vi "Enforce array size one timestamp.vi"(9 "#bytes per timestamp":i32, 11 "Values (new)":u8[](array[numeric])) -> (3 "Values (new) [padded]":u8[](array[numeric]))   [LabVIEW 2021, in "Ring Buffer Time Series Data.lvlib"]
doc: "This VIM will set a size to the <b>Array In</b> and pass it out as <b>Array Out</b>. This VIM can set a Minimum, or Maximum array size setting <b>Mode</b>. The size is then specified with <b>Size</b>. If elements need to be added or removed they can be processed to at the start of the array or the end. Returned will be the elements that needed to be added or removed to meet the size needs.\n\n-------------\nPackage Information\n\nProduct Name: Hooovahh Array VIMs\nPackage File Name: Hooovahh_Array_VIMs-2.1.1.12\nPackage Version: 2.1.1.12\nMinimum LabVIEW Version: 18.0"
uses:
  Ring Buffer Time Series Data.lvlib
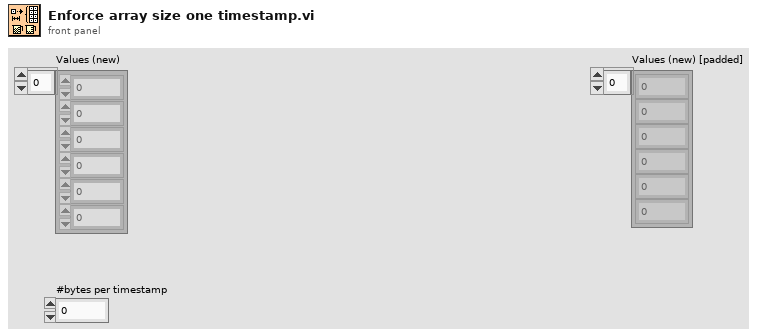
[diagram p1: front panel]
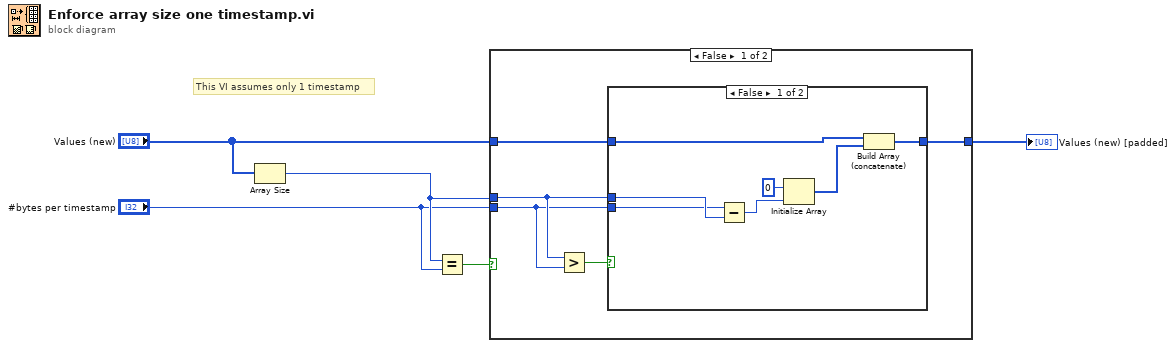
[diagram p0: block diagram]
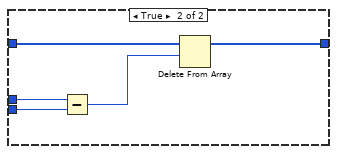
[diagram p2: hidden frame]
diagram:
  # "This VI assumes only 1 timestamp"
  n1 = Array Size(array="Values (new)") -> (size(s)=w3:i32)
  n2 = Equal?(x=w3, y="#bytes per timestamp") -> (x = y?=w2:bool)
  n3 = case shown="False" w2 {
    tunnel: "Values (new)" -> [w10 w23]
    tunnel: [w9 w23] -> w4
    tunnel: w3 -> [w7 _]
    tunnel: "#bytes per timestamp" -> [w6 _]
    frame False {
      n4 = Greater?(x=w7, y=w6) -> (0:w8:bool)
      n5 = case shown="False" w8 {
        tunnel: w7 -> [w16 w22]
        tunnel: w6 -> [w15 w21]
        tunnel: w10 -> [w12 w20]
        tunnel: [w14 w19] -> w9
        frame False {
          n6 = Subtract(x=w15, y=w16) -> (x-y=w17:i32)
          n7 = Initialize Array(u8 0 ("element"), w17) -> (w11:u8[])
          n8 = Build Array (concatenate)(w12, w11) -> (w14:u8[])
        }
        frame True {
          n9 = Subtract(x=w22, y=w21) -> (x-y=w18:i32)
          n10 = Delete From Array(array=w20, length=w18) -> (array with subset deleted=w19:u8[])  [unwired: 1 in, 1 out]
        }
      }
    }
    frame True {
    }
  }
  "Values (new) [padded]" <- w4
